vi "Prova QH H.vi"(4 "solo acquisizione!!":bool=TRUE, 6 "Text.Text":string="Prova QH: ", 7 "Tipo motore pompa":enum16{"Monofase", "Trifase"}(ring), 8 "Array % valvole":dbl[][](array[numeric]), 9 "Manuale F\\auto T":bool=TRUE, 10 "Status":refnum<vi>, 11 "input cluster":T1={"Scelta wattmetro"={"Wattmetro"=enum."No Selection"}, "SET RPM"=0.0, "SET TEMP"=0.0, "Array banchi"=[{"Nome"="Elettropompa", "Tors. scala1"=0, "Tors. scala2"=0, "rpm"=0, "TAMB"=0, "Indici Temperature"=[0, 1], "Indice freno"=1, "alimentatore trifase"=0, "alimentatore monofase"=0, "alimentatore dc arm"=0, "alimentatore dc ecc"=0, "alimentatore dc mp"=0}, {"Nome"="Sommersa", "Tors. scala1"=0, "Tors. scala2"=0, "rpm"=0, "TAMB"=1, "Indici Temperature"=[0, 1], "Indice freno"=0, "alimentatore trifase"=0, "alimentatore monofase"=0, "alimentatore dc arm"=0, "alimentatore dc ecc"=0, "alimentatore dc mp"=0}], "Array valvole linee avvio/fermata"=[], "banco selezionato"=0, "Nomi valvole prop sistema"=[], "canale-- sensore"=[], "Attriti B1"=[], "Attriti B2"=[], "Collegamento elettrico"={"ALIMENTAZIONE ELETTRICA"=enum."AC MONOFASE", "ID"=0, "#rami freddo\\eq term resmeter"=0, "#rami riscaldamento resmeter"=0, "#rami freddo\\eq term resistomat"=0, "#rami riscaldamento resistomat"=0, "CALCOLI"=enum."AC TRIFASE"}, "lingua"=0, "Costanti collaudo"={"P [bar]"=0.0, "T amb. [°C]"=0.0, "Umidità [%]"=0.0, "T acqua [°C] 2"=0.0}, "OPZIONI MISURE RES"={"MISURA A FREDDO"=enum."RESISTOMAT", "MISURA EQ. TERMICO"=enum."RESISTOMAT", "MISURA DT PROVA IN CORSO"=enum."RESISTOMAT - CON FERMATE", "MISURE PRIMA E DOPO"=enum."RESISTOMAT", "STRUMENTI PRESENTI"=enum."NESSUNO"}, "Dati targa motore"={"Vnom"=0.0, "Fnom"=0.0, "Inom"=0.0, "Cnom"=0.0, "Npoli"=0.0, "Scorta 1"=0.0, "Scorta 2"=0.0, "Scorta 3"=0.0}}) -> ()   [LabVIEW 2019]
uses:
  Tstabilizzazione auto.vi
  SubVI ELETTROTEST60A Folder/Elettrotest60A/Global_bypass_ResMeter.vi
  Ferma pompa auto.vi
  Global SETTINGS QH AUTO.vi
  TypeDef/WT SELECTION.ctl
  TypeDef/Definizione linea.ctl
  TypeDef/Cluster INFO.ctl
  TypeDef/Collegamenti_elettrici.ctl
  TypeDef/Control Calcoli.ctl
panel:
  out "Fine acq":bool
  in  "Reset":bool
  out "Set% valvole":dbl[](array[numeric])
  in  "Stato auto":string
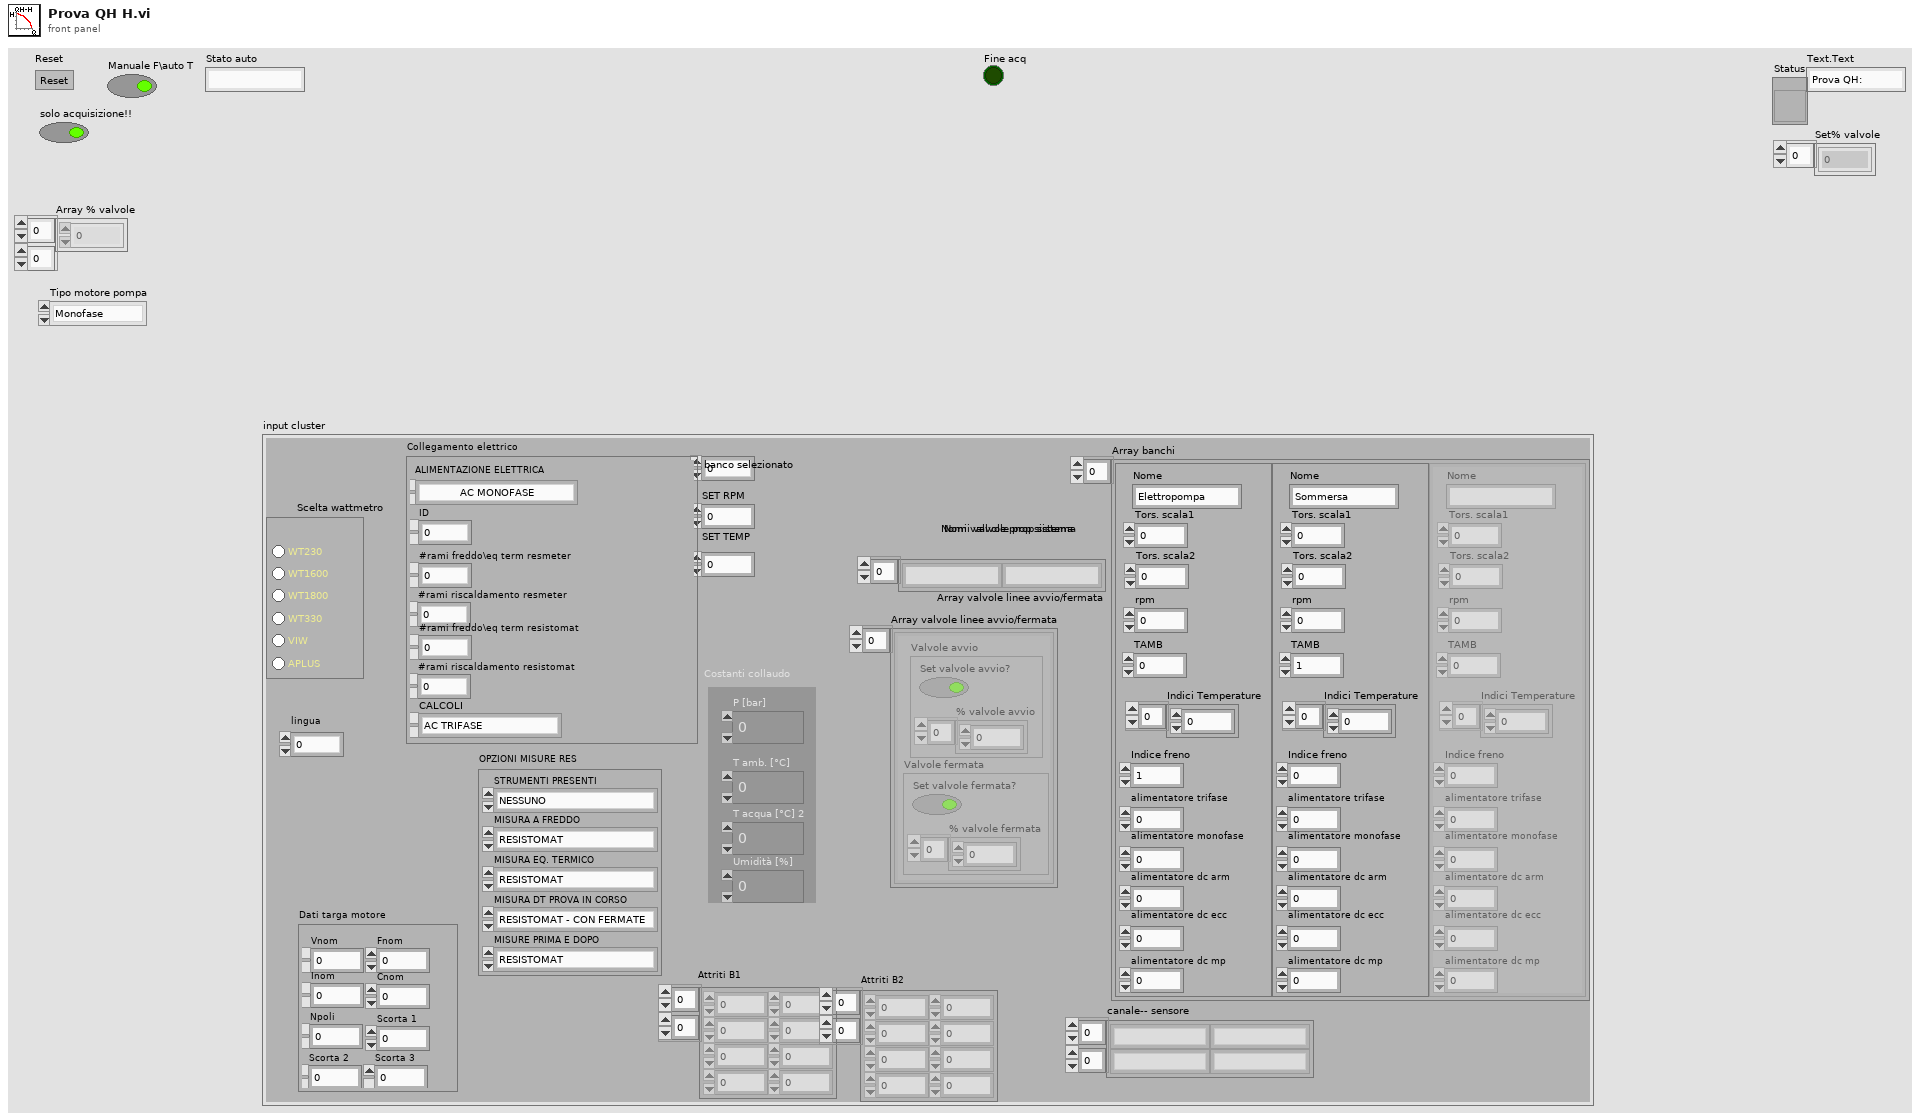
[diagram p1: front panel]
types:
  T1 = typedef "Cluster INFO.ctl" = cluster{"Scelta wattmetro":cluster{"Wattmetro":T2}, "SET RPM":dbl, "SET TEMP":dbl, "Array banchi":T3[], "Array valvole linee avvio/fermata":cluster{"Valvole avvio":cluster{"Set valvole avvio?":bool, "% valvole avvio":dbl[]}, "Valvole fermata":cluster{"Set valvole fermata?":bool, "% valvole fermata":dbl[]}}[], "banco selezionato":i8, "Nomi valvole prop sistema":string[], "canale-- sensore":string[][], "Attriti B1":dbl[][], "Attriti B2":dbl[][], "Collegamento elettrico":cluster{"ALIMENTAZIONE ELETTRICA":T4, "ID":i16, "#rami freddo\\eq term resmeter":i16, "#rami riscaldamento resmeter":i16, "#rami freddo\\eq term resistomat":i16, "#rami riscaldamento resistomat":i16, "CALCOLI":T5}, "lingua":i16, "Costanti collaudo":cluster{"P [bar]":dbl, "T amb. [°C]":dbl, "Umidità [%]":dbl, "T acqua [°C] 2":dbl}, "OPZIONI MISURE RES":cluster{"MISURA A FREDDO":enum16{"NESSUNO", "RESISTOMAT", "RES METER", "ENTRAMBI"}, "MISURA EQ. TERMICO":enum16{"NESSUNO", "RESISTOMAT", "RES METER", "ENTRAMBI"}, "MISURA DT PROVA IN CORSO":enum16{"NESSUNO", "RESISTOMAT - CON FERMATE", "RES METER - CON FERMATE", "RES METER - CONTINUO"}, "MISURE PRIMA E DOPO":enum16{"NESSUNO", "RESISTOMAT", "RES METER"}, "STRUMENTI PRESENTI":enum16{"NESSUNO", "RESISTOMAT", "RES METER", "ENTRAMBI"}}, "Dati targa motore":cluster{"Vnom":dbl, "Fnom":dbl, "Inom":dbl, "Cnom":dbl, "Npoli":dbl, "Scorta 1":dbl, "Scorta 2":dbl, "Scorta 3":dbl}}
  T2 = typedef "WT SELECTION.ctl" = enum32{"No Selection", "WT230", "WT1600", "WT1800", "WT330", "VIW", "APLUS"}
  T3 = typedef "Definizione linea.ctl" = cluster{"Nome":string, "Tors. scala1":i32, "Tors. scala2":i32, "rpm":i32, "TAMB":i32, "Indici Temperature":i16[], "Indice freno":i16, "alimentatore trifase":i16, "alimentatore monofase":i16, "alimentatore dc arm":i16, "alimentatore dc ecc":i16, "alimentatore dc mp":i16}
  T4 = typedef "Collegamenti_elettrici.ctl" = enum16{"AC TRIFASE", "AC TRIFASE + FRENO", "AC MONOFASE", "DC CON ECCITAZIONE", "DC CON ECCITAZIONE + FRENO", "DC NO ECCITAZIONE", "DC NO ECCITAZIONE + FRENO", "FRENO TRASC + AFE", "SOLO FRENO", "CARICO RESISTIVO", "GENERICO", "SOLO ACQUISITORE", "SCORTA 4", "SCORTA 5", "SCORTA 6"}
  T5 = typedef "Control Calcoli.ctl" = enum16{"AC TRIFASE", "AC MONOFASE", "DC ECCITAZIONE", "DC NO ECCITAZIONE", "POMPA TRIFASE", "POMPA MONOFASE", "GENERICO", "TRASFORMATORE", "ALTERNATORE TRASCINATO", "GRUPPO ELETTROGENO"}
  T6 = cluster{"Valvole avvio":cluster{"Set valvole avvio?":bool, "% valvole avvio":dbl[]}, "Valvole fermata":cluster{"Set valvole fermata?":bool, "% valvole fermata":dbl[]}}[]
  T7 = cluster{"Valvole avvio":cluster{"Set valvole avvio?":bool, "% valvole avvio":dbl[]}, "Valvole fermata":cluster{"Set valvole fermata?":bool, "% valvole fermata":dbl[]}}
  T8 = cluster{"Set valvole avvio?":bool, "% valvole avvio":dbl[]}
  T9 = cluster{"Set valvole fermata?":bool, "% valvole fermata":dbl[]}
  T10 = cluster{"Array of elements":cluster{"String":string, "variant":variant}[], "Single element":cluster{"String":string, "variant":variant}, "enque at\nopposite end (F)":bool, "no replications (F)":bool}
  T11 = cluster{"Durata risc. [min]":dbl, "Timer acq. [min]":dbl}
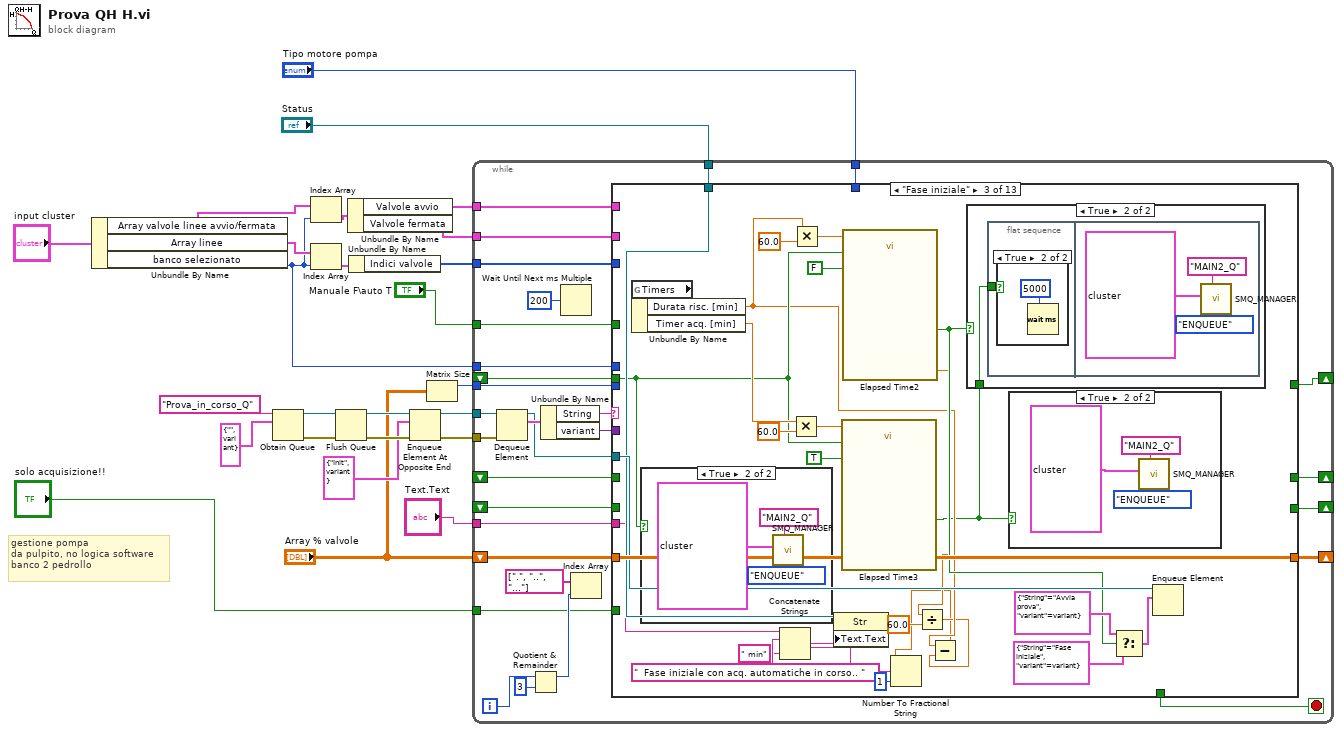
[diagram p0: block diagram]
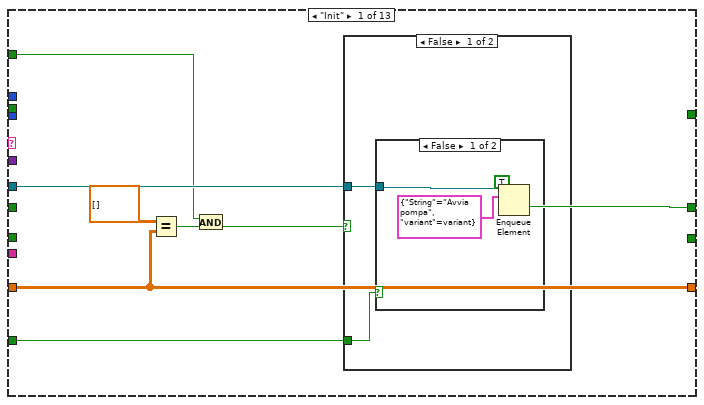
[diagram p2: hidden frame]
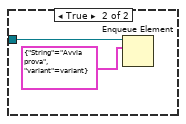
[diagram p3: hidden frame]
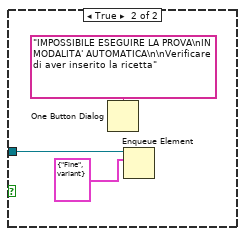
[diagram p4: hidden frame]
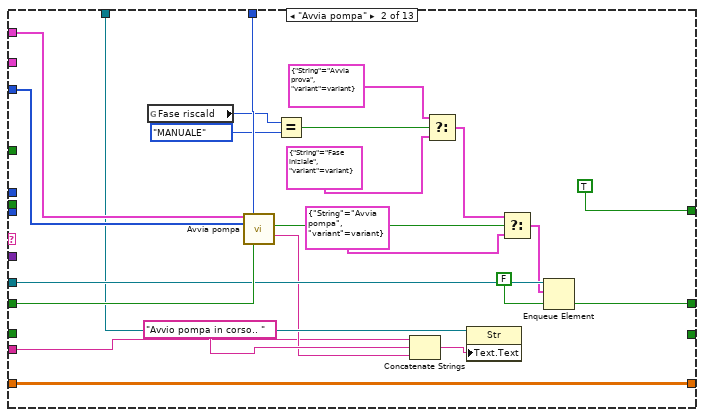
[diagram p5: hidden frame]
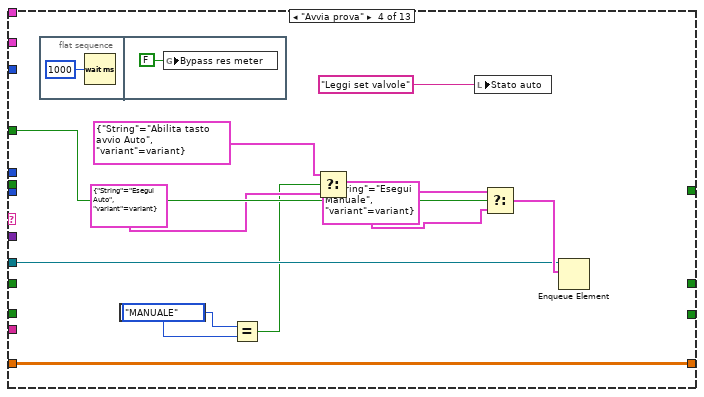
[diagram p10: hidden frame]
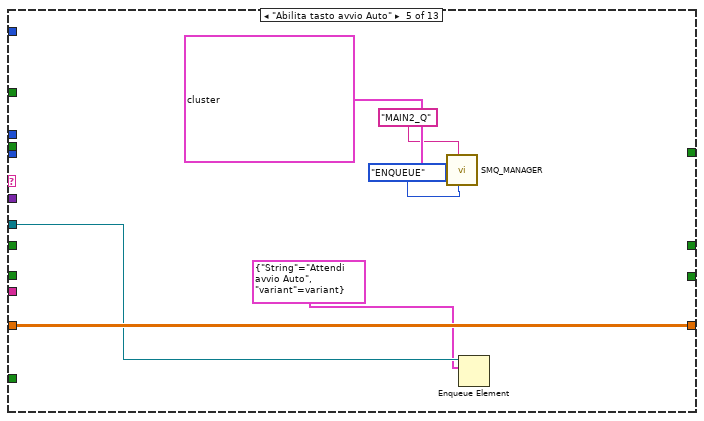
[diagram p11: hidden frame]
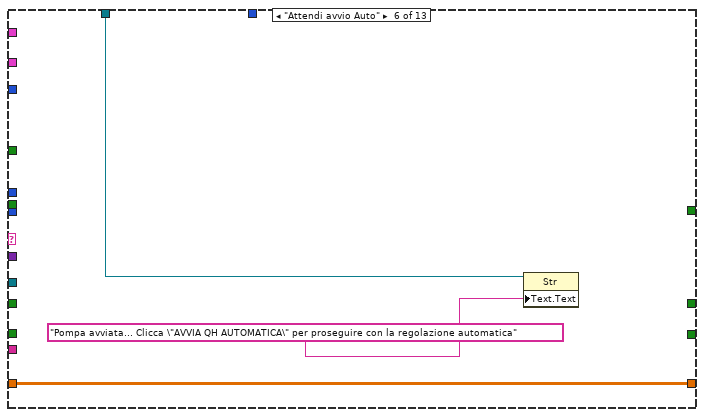
[diagram p12: hidden frame]
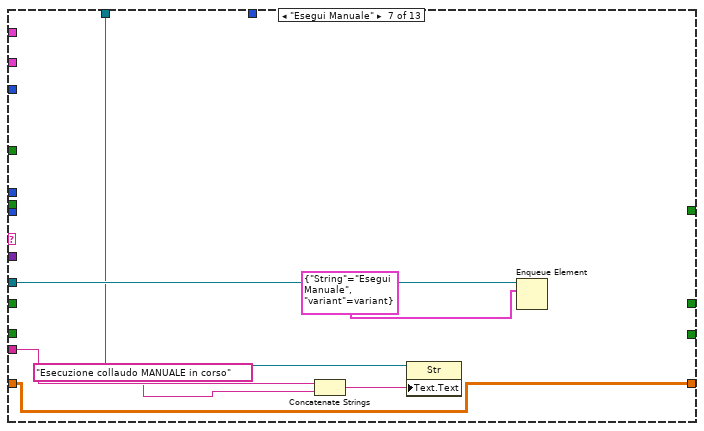
[diagram p13: hidden frame]
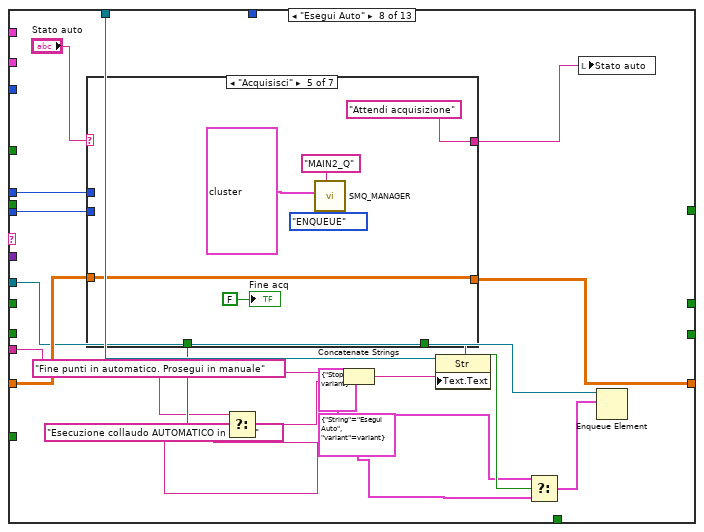
[diagram p14: hidden frame]
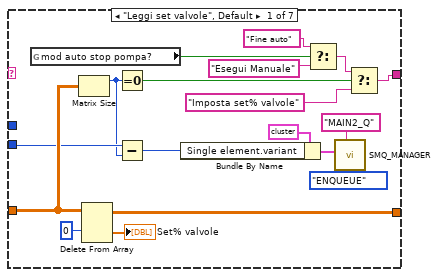
[diagram p15: hidden frame]
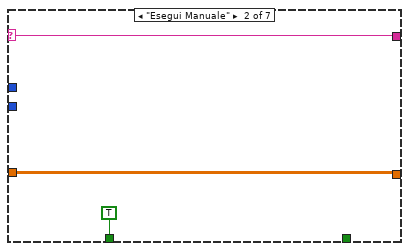
[diagram p16: hidden frame]
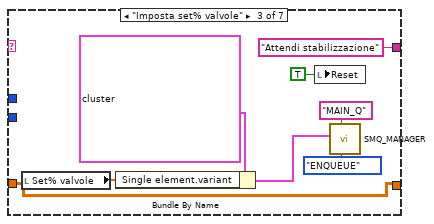
[diagram p17: hidden frame]
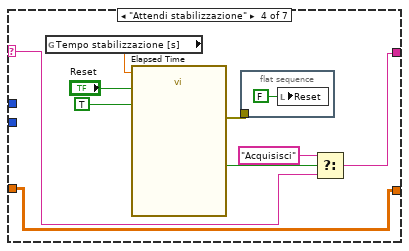
[diagram p18: hidden frame]
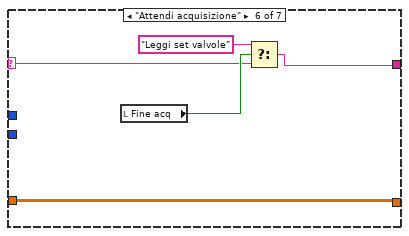
[diagram p19: hidden frame]
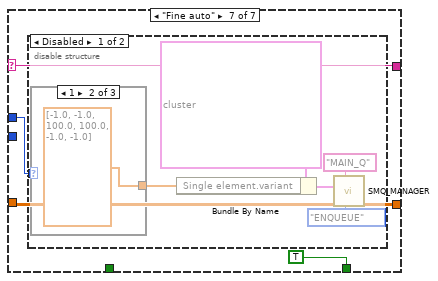
[diagram p20: hidden frame]
diagram:
  # "gestione pompa\nda pulpito, no logica software\nbanco 2 pedrollo"
  n1 = Unbundle By Name("input cluster") -> ("Array valvole linee avvio/fermata"=w12:T6, "Array linee"=w14:T3[], "banco selezionato"=w2:i8)
  n2 = Obtain Queue(name (unnamed)="Prova_in_corso_Q" ("Queue Name"), element data type=cluster{"String":string, "variant":variant} {"String"="", "variant"=variant} ("element")) -> (queue out=w19:refnum<queue>, error out=w18:errorcluster)  [unwired: 3 in, 1 out]
  n3 = Index Array(array=w12, index=w2) -> (element=w11:T7)
  n4 = Index Array(array=w14, index=w2) -> (element=w13:T3)
  n5 = Flush Queue(queue=w19, error in (no error)=w18) -> (queue out=w23:refnum<queue>, error out=w22:errorcluster)  [unwired: 1 out]
  n6 = Unbundle By Name(w11) -> ("Valvole avvio"=w9:T8, "Valvole fermata"=w8:T9)
  n7 = Unbundle By Name(w13) -> ("Indici valvole"=w7:i16[])
  n8 = Enqueue Element At Opposite End(queue=w23, element=cluster{"String":string, "variant":variant} {"String"="Init", "variant"=variant}, error in (no error)=w22) -> (queue out=w25:refnum<queue>, error out=w24:errorcluster)  [unwired: 1 in, 1 out]
  n9 = Matrix Size(0:"Array % valvole") -> (1:w3:i32)  [unwired: 1 out]
  n10 = while {
    tunnel: w25 -> [w55]
    tunnel: w24 -> [w54]
    tunnel: "Manuale F\\auto T" -> [w50]
    shift-right: [w49] -> _
    shift-left: "Array % valvole" -> [w48]
    shift-right: [w46] -> _
    shift-left: _ -> [w45]
    tunnel: w9 -> [w44]
    tunnel: "Tipo motore pompa" -> [w43]
    tunnel: w8 -> [w42]
    shift-right: [w41] -> _
    shift-left: _ -> [w40]
    tunnel: w7 -> [w39]
    tunnel: "Status" -> [w38]
    tunnel: "Text.Text" -> [w36]
    tunnel: w3 -> [w30]
    tunnel: "solo acquisizione!!" -> [w29]
    tunnel: w2 -> [w28]
    shift-right: [w27] -> _
    shift-left: _ -> [w26]
    i -> [w32]
    stop <- w37 stop-if-true
    n11 = Dequeue Element(queue=w55, error in (no error)=w54) -> (queue out=w47:refnum<queue>, element=w53:cluster{"String":string, "variant":variant})  [unwired: 1 in, 2 out]
    n12 = Quotient & Remainder(x=w32, y=3) -> (x-y*floor(x/y)=w35:i32)  [unwired: 1 out]
    n13 = Unbundle By Name(w53) -> ("String"=w52:string, "variant"=w51:variant)
    n14 = Wait Until Next ms Multiple(millisecond multiple=u32 200) -> ()  [unwired: 1 out]
    n15 = Index Array(array=string[] [".", "..", "..."], index=w35) -> ()  [unwired: 1 out]
    n16 = case shown="\"Fase iniziale\"" w52 {
      selector: w52 -> [_ _ _ _ _ _ _ _ _ _ _ _ w278]
      tunnel: w51 -> [_ _ _ _ _ _ _ _ _ _ _ _ _]
      tunnel: w50 -> [w57 _ _ w143 _ _ _ _ _ _ _ _ _]
      tunnel: [w63 w88 w122 w142 w154 w157 w158 w177 w247 w249 w257 w275 w279] -> w49
      tunnel: w48 -> [w63 w88 w122 w142 w154 w157 w158 w178 w247 w249 w257 w275 w279]
      tunnel: w47 -> [w60 w92 w114 w144 w153 _ w163 w175 _ w252 w266 _ _]
      tunnel: [TRUE FALSE _ _ _ _ _ _ _ _ w271 _ _] -> w46
      tunnel: w45 -> [_ w94 _ _ _ _ _ _ _ _ w271 _ _]
      tunnel: w44 -> [_ w86 _ _ _ _ _ _ _ _ _ _ _]
      tunnel: w43 -> [_ w87 _ _ _ _ _ _ _ _ w272 _ _]
      tunnel: w42 -> [_ _ _ _ _ _ _ _ _ _ w264 _ _]
      tunnel: [_ _ _ _ _ _ _ _ _ TRUE FALSE _ _] -> w41
      tunnel: w40 -> [_ _ _ _ _ _ _ _ _ _ w265 _ _]
      tunnel: w39 -> [_ w85 _ _ _ _ _ _ _ _ w263 _ _]
      tunnel: w38 -> [_ w84 w108 _ _ w156 w162 w181 _ _ w258 _ _]
      tunnel: [_ _ _ _ _ _ _ _ _ _ _ TRUE _] -> w37
      tunnel: w36 -> [_ w80 w106 _ _ _ w161 w180 _ _ w261 _ _]
      tunnel: w30 -> [_ _ _ _ _ _ _ w170 _ _ _ _ _]
      tunnel: w29 -> [w56 _ _ _ _ _ _ _ _ w248 _ _ _]
      tunnel: w28 -> [_ _ _ _ _ _ _ w169 _ _ _ _ _]
      tunnel: [_ TRUE _ _ _ _ _ _ _ _ _ _ _] -> w27
      tunnel: w26 -> [_ _ w104 _ _ _ _ _ _ _ _ _ _]
      frame "Init" {
        n17 = Equal?(x=dbl[][] [], y=w63) -> (x = y?=w61:bool)
        n18 = And(x=w57, y=w61) -> (x .and. y?=w58:bool)
        n19 = case shown="False" w58 {
          tunnel: w60 -> [w65 w71]
          tunnel: w56 -> [w64 _]
          frame False {
            n20 = case shown="False" w64 {
              tunnel: w65 -> [w66 w68]
              frame False {
                n21 = Enqueue Element(queue=w66, element=cluster{"String":string, "variant":variant} {"String"="Avvia pompa", "variant"=variant}) -> ()  [unwired: 2 in, 3 out]
              }
              frame True {
                n22 = Enqueue Element(queue=w68, element=cluster{"String":string, "variant":variant} {"String"="Avvia prova", "variant"=variant}) -> ()  [unwired: 2 in, 3 out]
              }
            }
          }
          frame True {
            n23 = One Button Dialog(message="IMPOSSIBILE ESEGUIRE LA PROVA\nIN MODALITA' AUTOMATICA\n\nVerificare di aver inserito la ricetta") -> ()  [unwired: 1 in, 1 out]
            n24 = Enqueue Element(queue=w71, element=cluster{"String":string, "variant":variant} {"String"="Fine", "variant"=variant}) -> ()  [unwired: 2 in, 3 out]
          }
        }
      }
      frame "Avvia pompa" {
        n25 = global read "Global SETTINGS QH AUTO.vi" "Fase riscald"() -> (w79:enum32{"MANUALE", "AUTO TIMER"})
        n26 = call "Avvia pompa.vi"("Valvole avvio"=w86, "Tipo motore pompa"=w87, "Indici valvole linea"=w85, "Reset avvio"=w94) -> ("Fine Avvio"=w91:bool, "stato"=w81:string)  [unwired: 10 in]
        n27 = Equal?(x=w79, y=enum32{"MANUALE", "AUTO TIMER"}."MANUALE") -> (x = y?=w77:bool)
        n28 = Concatenate Strings(w80, "Avvio pompa in corso.. " ("Text.Text"), w81) -> (w82:string)
        n29 = Select(t=cluster{"String":string, "variant":variant} {"String"="Avvia prova", "variant"=variant} ("element"), s=w77, f=cluster{"String":string, "variant":variant} {"String"="Fase iniziale", "variant"=variant} ("element")) -> (s? t:f=w75:cluster{"String":string, "variant":variant})
        n30 = property class="Str"(reference=w84, "Text.Text"=w82) -> ()  [unwired: 1 in, 2 out]
        n31 = Select(t=w75, s=w91, f=cluster{"String":string, "variant":variant} {"String"="Avvia pompa", "variant"=variant} ("element")) -> (s? t:f=w89:cluster{"String":string, "variant":variant})
        n32 = Enqueue Element(queue=w92, element=w89) -> ()  [unwired: 2 in, 3 out]
      }
      frame "Fase iniziale" {
        n33 = global read "Global SETTINGS QH AUTO.vi" "Timers"() -> (w121:T11)
        n34 = Unbundle By Name(w121) -> ("Durata risc. [min]"=w101:dbl, "Timer acq. [min]"=w116:dbl)
        n35 = case shown="True" w104 {
          frame False {
          }
          frame True {
            n36 = call <userlib>:"SMQ_MANAGER.vi"("Function"=enum16{"INITIALIZE", "ENQUEUE", "STOP ALL"}."ENQUEUE", "Queue name"="MAIN2_Q", "Enqueue cluster"=T10 {"Array of elements"=[], "Single element"={"String"="SCELTA TAB2", "variant"=variant}, "enque at\nopposite end (F)"=FALSE, "no replications (F)"=FALSE}) -> ()  [unwired: 8 in, 1 out]
          }
        }
        n37 = Multiply(x=w116, y=60.0) -> (x*y=w118:dbl)
        n38 = Multiply(x=w101, y=60.0) -> (x*y=w119:dbl)
        n39 = call "Elapsed Time3"("Time Target (s)"=w118, "Reset"=w104, "Auto Reset"=TRUE) -> ("Time has Elapsed"=w95:bool)  [unwired: 9 in, 7 out]
        n40 = call "Elapsed Time2"("Time Target (s)"=w119, "Reset"=w104, "Auto Reset"=FALSE) -> ("Elapsed Time (s)"=w103:dbl, "Time has Elapsed"=w109:bool)  [unwired: 9 in, 6 out]
        n41 = Divide(x=w103, y=60.0) -> (x/y=w100:dbl)
        n42 = Subtract(x=w101, y=w100) -> (x-y=w99:dbl)
        n43 = Number To Fractional String(number=w99, precision (6)=i16 1) -> (F-format string=w97:string)  [unwired: 2 in]
        n44 = Concatenate Strings(w106, "  Fase iniziale con acq. automatiche in corso.. " ("string"), w97, " min" ("string")) -> (w107:string)
        n45 = property class="Str"(reference=w108, "Text.Text"=w107) -> ()  [unwired: 1 in, 2 out]
        n46 = case shown="True" w109 {
          tunnel: w95 -> [_ w126]
          frame False {
          }
          frame True {
            n47 = flat-sequence {
              tunnel: w126 -> [w127]
              frame #0 {
                n48 = case shown="True" w127 {
                  frame False {
                  }
                  frame True {
                    n49 = Wait (ms)(milliseconds to wait=u32 5000) -> ()  [unwired: 1 out]
                  }
                }
              }
              frame #1 {
                n50 = call <userlib>:"SMQ_MANAGER.vi"("Function"=enum16{"INITIALIZE", "ENQUEUE", "STOP ALL"}."ENQUEUE", "Queue name"="MAIN2_Q", "Enqueue cluster"=T10 {"Array of elements"=[], "Single element"={"String"="SCELTA TAB1", "variant"=variant}, "enque at\nopposite end (F)"=FALSE, "no replications (F)"=FALSE}) -> ()  [unwired: 8 in, 1 out]
              }
            }
          }
        }
        n51 = case shown="True" w95 {
          frame False {
          }
          frame True {
            n52 = call <userlib>:"SMQ_MANAGER.vi"("Function"=enum16{"INITIALIZE", "ENQUEUE", "STOP ALL"}."ENQUEUE", "Queue name"="MAIN2_Q", "Enqueue cluster"=T10 {"Array of elements"=[], "Single element"={"String"="AQ AUTO", "variant"=variant}, "enque at\nopposite end (F)"=FALSE, "no replications (F)"=FALSE}) -> ()  [unwired: 8 in, 1 out]
          }
        }
        n53 = Select(t=cluster{"String":string, "variant":variant} {"String"="Avvia prova", "variant"=variant} ("element"), s=w109, f=cluster{"String":string, "variant":variant} {"String"="Fase iniziale", "variant"=variant} ("element")) -> (s? t:f=w112:cluster{"String":string, "variant":variant})
        n54 = Enqueue Element(queue=w114, element=w112) -> ()  [unwired: 2 in, 3 out]
      }
      frame "Avvia prova" {
        n55 = flat-sequence {
          frame #0 {
            n56 = Wait (ms)(milliseconds to wait=u32 1000) -> ()  [unwired: 1 out]
          }
          frame #1 {
            n57 = global write "Global_bypass_ResMeter.vi" "Bypass res meter"(FALSE ("Bypass res meter")) -> ()
          }
        }
        n58 = global read "Global SETTINGS QH AUTO.vi" "Fase riscald"() -> (w140:enum32{"MANUALE", "AUTO TIMER"})
        n59 = Equal?(x=w140, y=enum32{"MANUALE", "AUTO TIMER"}."MANUALE") -> (x = y?=w135:bool)
        n60 = Select(t=cluster{"String":string, "variant":variant} {"String"="Abilita tasto avvio Auto", "variant"=variant} ("element"), s=w135, f=cluster{"String":string, "variant":variant} {"String"="Esegui Auto", "variant"=variant}) -> (s? t:f=w137:cluster{"String":string, "variant":variant})
        n61 = local write "Stato auto"("Leggi set valvole" ("Stato auto")) -> ()
        n62 = Select(t=w137, s=w143, f=cluster{"String":string, "variant":variant} {"String"="Esegui Manuale", "variant"=variant} ("element")) -> (s? t:f=w145:cluster{"String":string, "variant":variant})
        n63 = Enqueue Element(queue=w144, element=w145) -> ()  [unwired: 2 in, 3 out]
      }
      frame "Abilita tasto avvio Auto" {
        n64 = call <userlib>:"SMQ_MANAGER.vi"("Function"=enum16{"INITIALIZE", "ENQUEUE", "STOP ALL"}."ENQUEUE", "Queue name"="MAIN2_Q", "Enqueue cluster"=T10 {"Array of elements"=[], "Single element"={"String"="ABILITA TASTO AVVIO AUTO", "variant"=variant}, "enque at\nopposite end (F)"=FALSE, "no replications (F)"=FALSE}) -> ()  [unwired: 8 in, 1 out]
        n65 = Enqueue Element(queue=w153, element=cluster{"String":string, "variant":variant} {"String"="Attendi avvio Auto", "variant"=variant}) -> ()  [unwired: 2 in, 3 out]
      }
      frame "Attendi avvio Auto" {
        n66 = property class="Str"(reference=w156, "Text.Text"="Pompa avviata... Clicca \"AVVIA QH AUTOMATICA\" per proseguire con la regolazione automatica") -> ()  [unwired: 1 in, 2 out]
      }
      frame "Esegui Manuale" {
        n67 = Concatenate Strings(w161, "Esecuzione collaudo MANUALE in corso" ("string")) -> (w160:string)
        n68 = property class="Str"(reference=w162, "Text.Text"=w160) -> ()  [unwired: 1 in, 2 out]
        n69 = Enqueue Element(queue=w163, element=cluster{"String":string, "variant":variant} {"String"="Esegui Manuale", "variant"=variant}) -> ()  [unwired: 2 in, 3 out]
      }
      frame "Esegui Auto" {
        n70 = case shown="\"Acquisisci\"" "Stato auto" {
          selector: "Stato auto" -> [_ w203 _ w215 _ w231 w236]
          tunnel: w178 -> [w197 w202 w204 w212 w222 w228 w235]
          tunnel: [w199 w202 w204 w212 w222 w228 w235] -> w177
          tunnel: [w194 w203 "Attendi stabilizzazione" w214 "Attendi acquisizione" ("t") w230 w236] -> w176
          tunnel: [_ _ _ _ _ _ TRUE] -> w172
          tunnel: w170 -> [w193 _ _ _ _ _ _]
          tunnel: w169 -> [_ _ _ _ _ _ w234]
          tunnel: [_ TRUE _ _ _ _ _] -> w167
          frame "Leggi set valvole", Default {
            n71 = global read "Ferma pompa auto.vi" "mod auto stop pompa?"() -> (w184:bool)
            n72 = Matrix Size(0:w197) -> (1:w192:i32)  [unwired: 1 out]
            n73 = Delete From Array(array=w197, index (row)=0) -> (deleted portion=→"Set% valvole":dbl[], array with subset deleted=w199:dbl[][])  [unwired: 2 in]
            n74 = Equal To 0?(x=w192) -> (x = 0?=w196:bool)
            n75 = Subtract(x=w193, y=w192) -> (x-y=w187:i32)
            n76 = Bundle By Name(cluster=T10 {"Array of elements"=[], "Single element"={"String"="PUNTO QH AUTO", "variant"=variant}, "enque at\nopposite end (F)"=FALSE, "no replications (F)"=FALSE} ("Enqueue cluster"), "Single element.variant"=w187) -> (w191:T10)
            n77 = Select(t="Fine auto", s=w184, f="Esegui Manuale") -> (s? t:f=w185:string)
            n78 = call <userlib>:"SMQ_MANAGER.vi"("Function"=enum16{"INITIALIZE", "ENQUEUE", "STOP ALL"}."ENQUEUE", "Queue name"="MAIN2_Q", "Enqueue cluster"=w191) -> ()  [unwired: 8 in, 1 out]
            n79 = Select(t=w185, s=w196, f="Imposta set% valvole") -> (s? t:f=w194:string)
          }
          frame "Esegui Manuale" {
          }
          frame "Imposta set% valvole" {
            n80 = local read "Set% valvole"() -> (w207:dbl[])
            n81 = Bundle By Name(cluster=T10 {"Array of elements"=[], "Single element"={"String"="COMANDI VALVOLE PROP", "variant"=variant}, "enque at\nopposite end (F)"=FALSE, "no replications (F)"=FALSE} ("Enqueue cluster"), "Single element.variant"=w207) -> (w211:T10)
            n82 = local write "Reset"(TRUE ("Reset")) -> ()
            n83 = call <userlib>:"SMQ_MANAGER.vi"("Function"=enum16{"INITIALIZE", "ENQUEUE", "STOP ALL"}."ENQUEUE", "Queue name"="MAIN_Q", "Enqueue cluster"=w211) -> ()  [unwired: 8 in, 1 out]
          }
          frame "Attendi stabilizzazione" {
            n84 = global read "Tstabilizzazione auto.vi" "Tempo stabilizzazione [s]"() -> (w217:dbl)
            n85 = call "Elapsed Time"("Time Target (s)"=w217, "Reset"="Reset", "Auto Reset"=TRUE) -> ("Time has Elapsed"=w216:bool, "error out"=w218:errorcluster)  [unwired: 9 in, 6 out]
            n86 = flat-sequence {
              tunnel: w218 -> [_]
              frame #0 {
                n87 = local write "Reset"(FALSE ("Reset")) -> ()
              }
            }
            n88 = Select(t="Acquisisci", s=w216, f=w215) -> (s? t:f=w214:string)
          }
          frame "Acquisisci" {
            n89 = call <userlib>:"SMQ_MANAGER.vi"("Function"=enum16{"INITIALIZE", "ENQUEUE", "STOP ALL"}."ENQUEUE", "Queue name"="MAIN2_Q", "Enqueue cluster"=T10 {"Array of elements"=[], "Single element"={"String"="AQ AUTO", "variant"=variant}, "enque at\nopposite end (F)"=FALSE, "no replications (F)"=FALSE}) -> ()  [unwired: 8 in, 1 out]
            "Fine acq" <- FALSE
          }
          frame "Attendi acquisizione" {
            n90 = local read "Fine acq"() -> (w232:bool)
            n91 = Select(t="Leggi set valvole", s=w232, f=w231) -> (s? t:f=w230:string)
          }
          frame "Fine auto" {
            n92 = disable-structure shown="Disabled" {
              disable-tunnel: w234 -> [w238 _]
              frame Disabled {
                n93 = case shown="1" w238 {
                  tunnel: [dbl[] [100.0, 100.0, -1.0, -1.0, -1.0, -1.0] dbl[] [-1.0, -1.0, 100.0, 100.0, -1.0, -1.0] dbl[] [-1.0, -1.0, -1.0, -1.0, 100.0, 100.0]] -> w237
                  frame 0, Default {
                  }
                  frame 1 {
                  }
                  frame 2 {
                  }
                }
                n94 = Bundle By Name(cluster=T10 {"Array of elements"=[], "Single element"={"String"="COMANDI VALVOLE PROP", "variant"=variant}, "enque at\nopposite end (F)"=FALSE, "no replications (F)"=FALSE} ("Enqueue cluster"), "Single element.variant"=w237) -> (w242:T10)
                n95 = call <userlib>:"SMQ_MANAGER.vi"("Function"=enum16{"INITIALIZE", "ENQUEUE", "STOP ALL"}."ENQUEUE", "Queue name"="MAIN_Q", "Enqueue cluster"=w242) -> ()  [unwired: 8 in, 1 out]
              }
              frame Enabled {
              }
            }
          }
        }
        n96 = Select(t="Fine punti in automatico. Prosegui in manuale" ("string"), s=w167, f="Esecuzione collaudo AUTOMATICO in corso" ("string")) -> (s? t:f=w165:string)
        n97 = Concatenate Strings(w180, w165) -> (w182:string)
        n98 = property class="Str"(reference=w181, "Text.Text"=w182) -> ()  [unwired: 1 in, 2 out]
        n99 = Select(t=cluster{"String":string, "variant":variant} {"String"="Stop", "variant"=variant} ("element"), s=w172, f=cluster{"String":string, "variant":variant} {"String"="Esegui Auto", "variant"=variant} ("element")) -> (s? t:f=w173:cluster{"String":string, "variant":variant})
        n100 = local write "Stato auto"(w176) -> ()
        n101 = Enqueue Element(queue=w175, element=w173) -> ()  [unwired: 2 in, 3 out]
      }
      frame "FINE ACQ" {
        n102 = local write "Fine acq"(TRUE ("Fine acq")) -> ()
      }
      frame "Stop" {
        n103 = Flush Queue(queue=w252) -> (queue out=w251:refnum<queue>)  [unwired: 1 in, 2 out]
        n104 = case shown="False" w248 {
          tunnel: w251 -> [w253 w255]
          frame False {
            n105 = Enqueue Element(queue=w253, element=cluster{"String":string, "variant":variant} {"String"="Ferma pompa", "variant"=variant}) -> ()  [unwired: 2 in, 3 out]
          }
          frame True {
            n106 = Enqueue Element(queue=w255, element=cluster{"String":string, "variant":variant} {"String"="Fine", "variant"=variant}) -> ()  [unwired: 2 in, 3 out]
          }
        }
      }
      frame "Ferma pompa" {
        n107 = call "Ferma pompa.vi"("Reset fermata"=w265, "Tipo motore pompa"=w272, "Indici valvole linea"=w263, "Valvole fermata"=w264) -> ("stato"=w259:string, "Fine Fermata"=w267:bool)  [unwired: 6 in]
        n108 = Concatenate Strings(w261, "Arresto pompa in corso... " ("string"), w259) -> (w262:string)
        n109 = property class="Str"(reference=w258, "Text.Text"=w262) -> ()  [unwired: 1 in, 2 out]
        n110 = Select(t=cluster{"String":string, "variant":variant} {"String"="Fine", "variant"=variant} ("element"), s=w267, f=cluster{"String":string, "variant":variant} {"String"="Ferma pompa", "variant"=variant} ("element")) -> (s? t:f=w269:cluster{"String":string, "variant":variant})
        n111 = Enqueue Element(queue=w266, element=w269) -> ()  [unwired: 2 in, 3 out]
      }
      frame "Fine" {
      }
      frame "CASE INESISTENTE", Default {
        n112 = Concatenate Strings(w278, " CASE INESISTENTE" ("string")) -> (w277:string)
        n113 = One Button Dialog(message=w277) -> ()  [unwired: 1 in, 1 out]
      }
    }
  }
